vi "Main.vi"() -> ()   [LabVIEW 2018]
uses:
  C:/GIT/gaialabviewclient/Gaia_LabVIEW/Resources/JOT.GaiaClient.dll
  Gaia_LabVIEW/Resources/JOT.GaiaClient.dll
  Typedefs/States.ctl
  Typedefs/Element.ctl
  Typedefs/TestSequence.ctl
panel:
  out "EventLog":string="\r\n"
  out "ClientConnection":bool
  out "StateEnum":T1
  in  "baseUrl":string="http://172.23.225.64 "
  out "error out":errorcluster
  in  "Exit":bool
  in  "Tab Control":enum32{"TestSequense", "ManualControls"}(tab)
  in  "TestSeqMode":bool
  out "TestSequenceState":T2=enum."WaitDUT"
  in  "Recover":bool
  in  "Release":bool
  in  "Slide":bool
  in  "BatteryConnector":bool
  # "Stateful Applications"
  # "Triggers"
  # "More StateApp manual controls \ncan be added here"
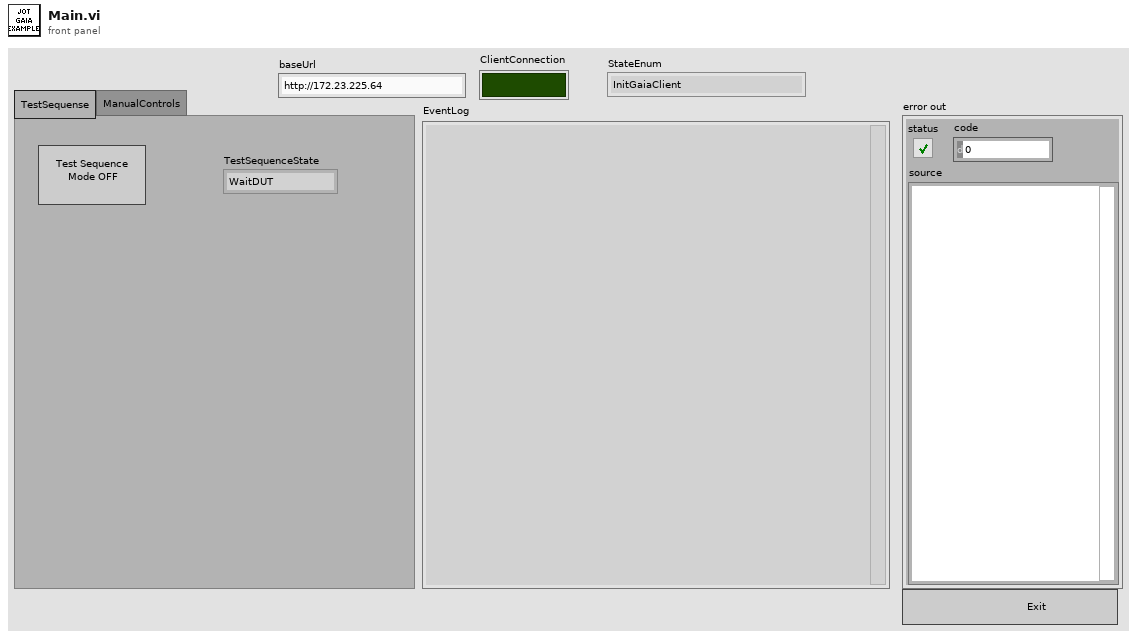
[diagram p1: front panel]
types:
  T1 = typedef "States.ctl" = enum16{"InitGaiaClient", "Idle", "AppsManualCtr", "StateTriggers", "TestSequence", "Exit"}
  T2 = typedef "TestSequence.ctl" = enum16{"SimulateDUTReplacement", "WaitDUT", "WaitReadyForTesting", "Test1", "ReleaseDUT"}
  T3 = typedef "Element.ctl" = cluster{"State":T1, "Application":string, "Action":string, "G code":string}
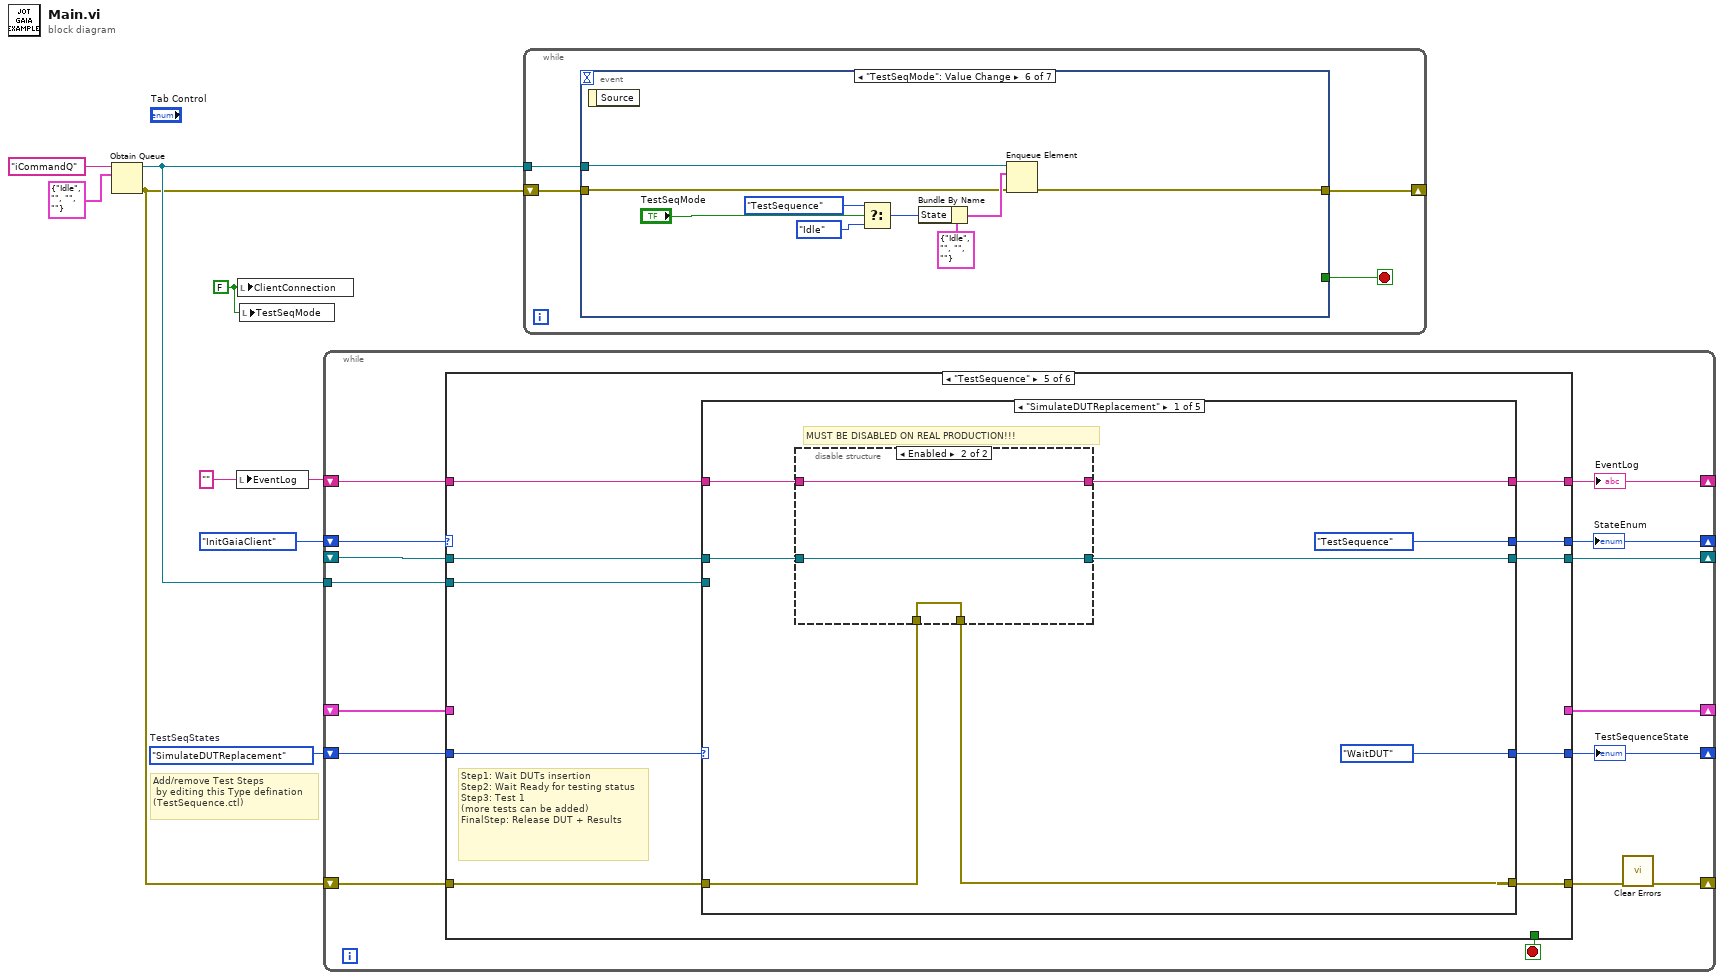
[diagram p0: block diagram]
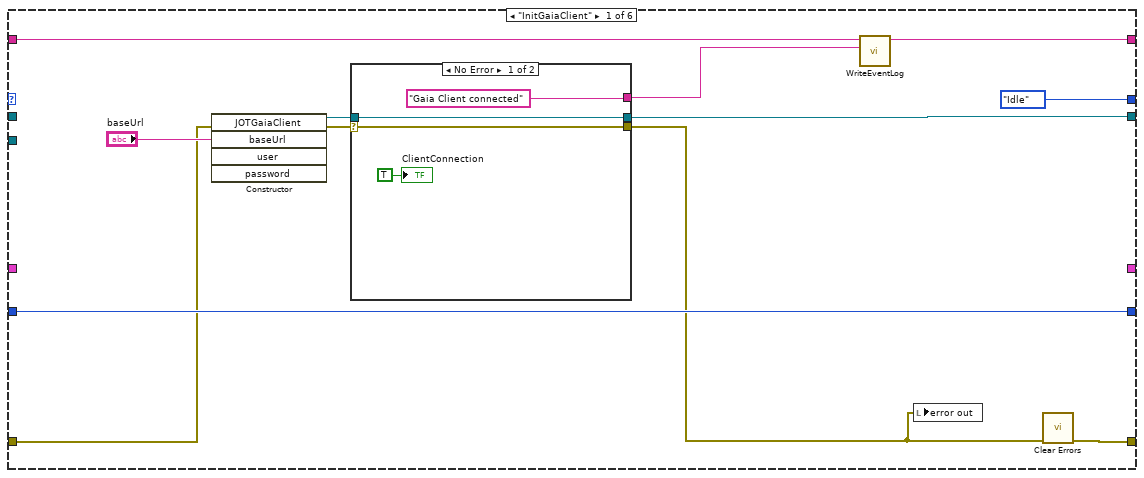
[diagram p2: hidden frame]
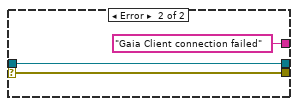
[diagram p3: hidden frame]
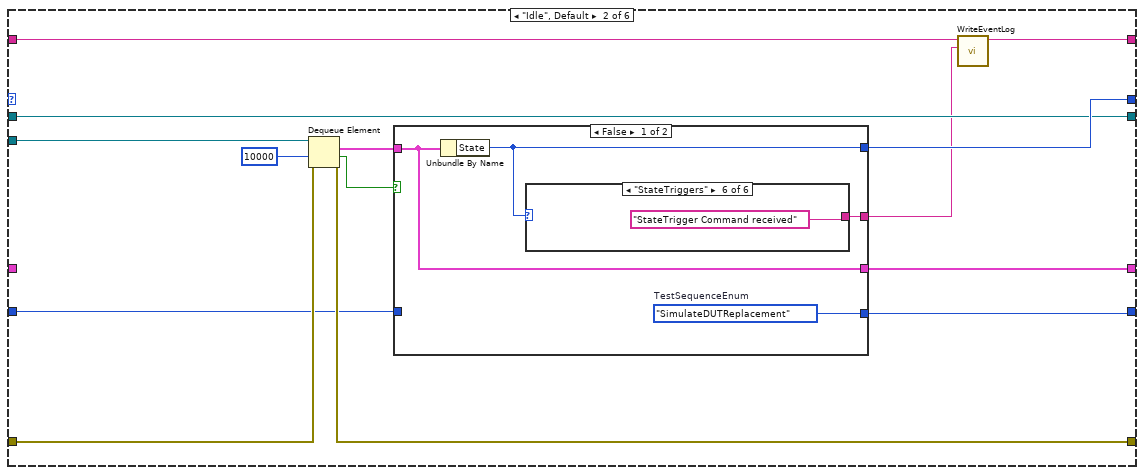
[diagram p4: hidden frame]
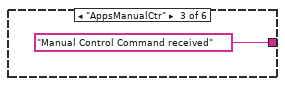
[diagram p7: hidden frame]
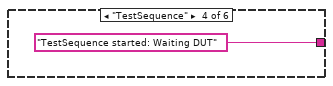
[diagram p8: hidden frame]
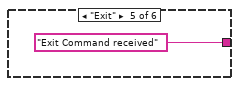
[diagram p9: hidden frame]
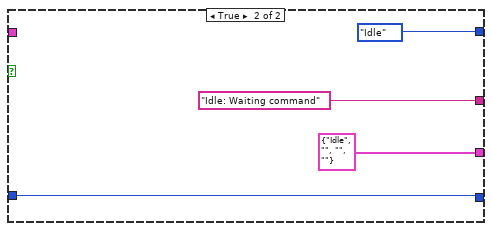
[diagram p10: hidden frame]
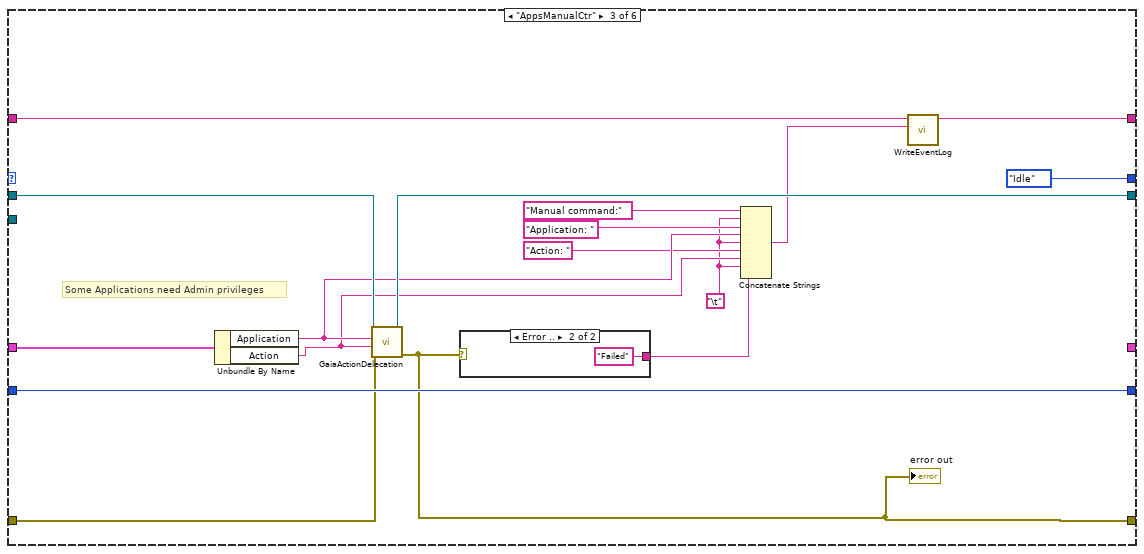
[diagram p11: hidden frame]
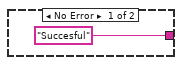
[diagram p12: hidden frame]
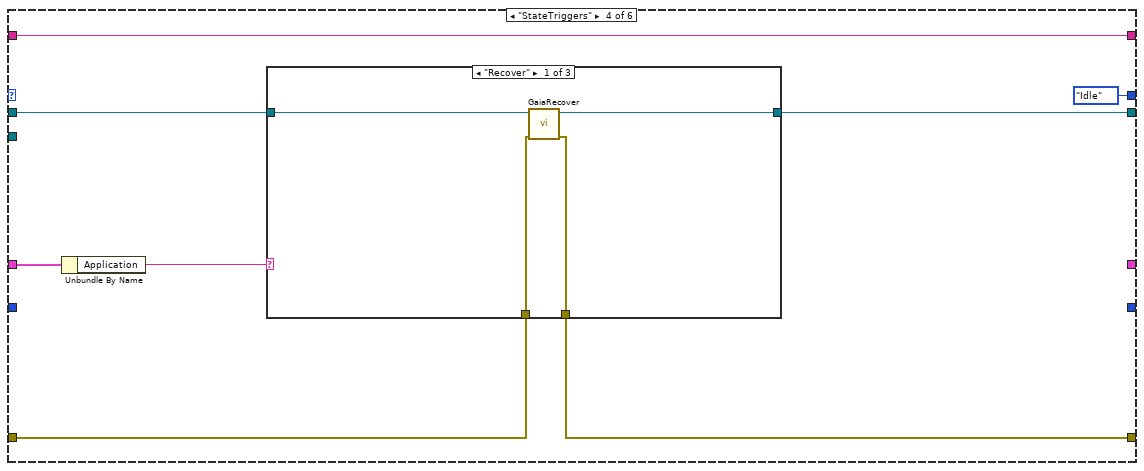
[diagram p13: hidden frame]
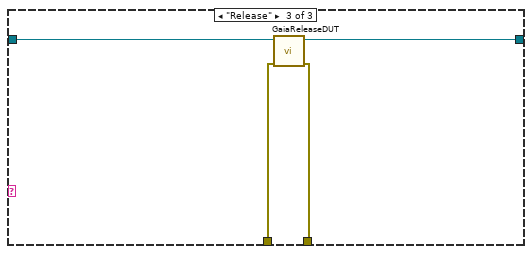
[diagram p15: hidden frame]
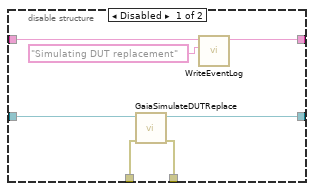
[diagram p16: hidden frame]
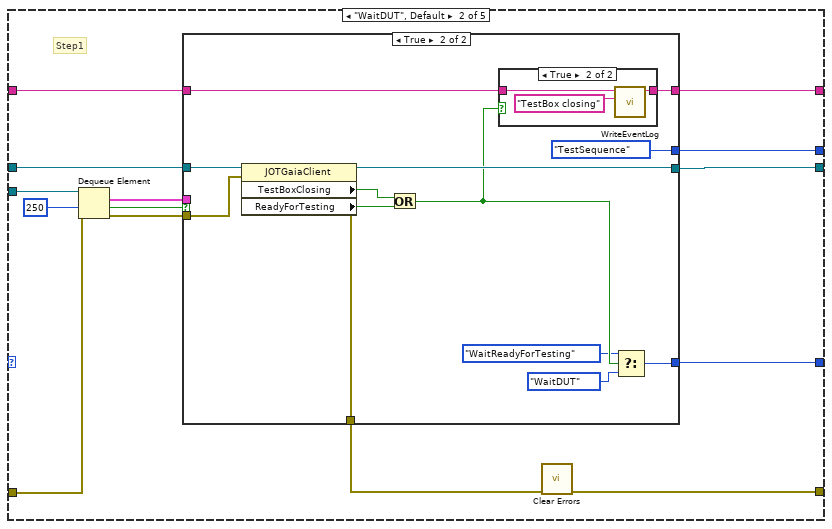
[diagram p17: hidden frame]
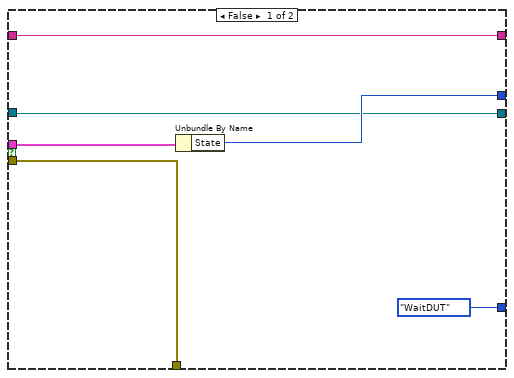
[diagram p18: hidden frame]
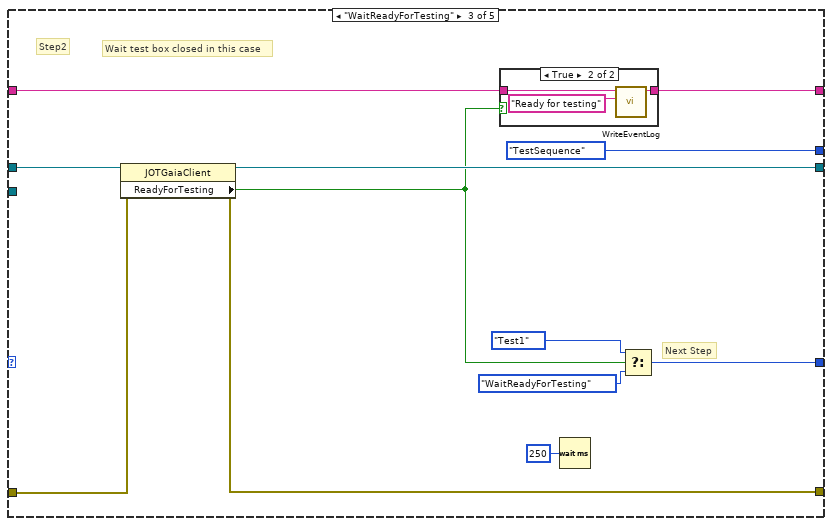
[diagram p20: hidden frame]
diagram:
  w1 = FALSE ("ClientConnection")
  w2 = ""
  w4 = TestSequence."SimulateDUTReplacement"  # TestSeqStates
  # "Add/remove Test Steps\n by editing this Type defination\n(TestSequence.ctl)"
  n1 = Obtain Queue(name (unnamed)="iCommandQ", element data type=T3 {"State"=enum."Idle", "Application"="", "Action"="", "G code"=""}) -> (queue out=w5:refnum<queue>, error out=w3:errorcluster)  [unwired: 3 in, 1 out]
  n2 = local write "EventLog"(w2) -> ()
  n3 = local write "ClientConnection"(w1) -> ()
  n4 = local write "TestSeqMode"(w1) -> ()
  n5 = while {
    shift-right: [w13] -> _
    shift-left: States."InitGaiaClient" -> [w23]
    shift-right: [w22] -> _
    shift-left: _ -> [w16]
    shift-right: [w10] -> _
    shift-left: w3 -> [w20]
    tunnel: w5 -> [w19]
    shift-right: [w18] -> _
    shift-left: _ -> [w17]
    shift-right: [w14] -> _
    shift-left: w4 -> [w15]
    shift-right: [w11] -> _
    shift-left: w2 -> [w12]
    stop <- w21 stop-if-true
    n6 = case shown="\"TestSequence\"" w23 {
      tunnel: [_ _ _ _ _ TRUE] -> w21
      tunnel: [w29 w49 w81 w89 w114 _] -> w22
      tunnel: w20 -> [w30 w54 w80 w93 w111 w224]
      tunnel: [w24 w55 w69 w91 w110 w218] -> w9
      tunnel: [States."Idle" w50 States."Idle" States."Idle" w108 States."Exit"] -> w13
      tunnel: w19 -> [_ w53 _ _ w109 w227]
      tunnel: [_ w48 _ _ _ _] -> w18
      tunnel: w17 -> [_ _ w84 w92 _ _]
      tunnel: w16 -> [_ w49 w82 w94 w115 w230]
      tunnel: w15 -> [w32 w46 w83 _ w113 w228]
      tunnel: [w32 w47 w83 _ w112 w228] -> w14
      tunnel: w12 -> [w28 w45 w79 w95 w107 w222]
      tunnel: [w27 w44 w78 w95 w106 w221] -> w11
      frame "InitGaiaClient" {
        n7 = constructor class="JOTGaiaClient"(error in=w30, "baseUrl"="baseUrl") -> (reference out=w34:refnum<k24>, error out=w31:errorcluster)  [unwired: 4 in, 4 out]
        n8 = case shown="No Error" w31 {
          selector: w31 -> [w37 w42]
          tunnel: w34 -> [w39 w41]
          tunnel: [w37 w42] -> w25
          tunnel: [w39 w41] -> w29
          tunnel: ["Gaia Client connected" ("LogText") "Gaia Client connection failed" ("LogText")] -> w26
          frame No Error {
            "ClientConnection" <- TRUE ("ClientConnection")
          }
          frame Error {
          }
        }
        n9 = call "WriteEventLog.vi"("LogText"=w26, "EventLog"=w28) -> ("EventLogOut"=w27:string)  [unwired: 9 in]
        n10 = local write "error out"(w25) -> ()
        n11 = call <vilib>:"Clear Errors.vi"("error in (no error)"=w25) -> ("error out"=w24:errorcluster)  [unwired: 5 in, 1 out]
      }
      frame "Idle", Default {
        n12 = Dequeue Element(queue=w53, timeout in ms (-1)=10000, error in (no error)=w54) -> (element=w56:T3, timed out?=w51:bool, error out=w55:errorcluster)  [unwired: 1 out]
        n13 = case shown="False" w51 {
          tunnel: w56 -> [w60 _]
          tunnel: [w58 States."Idle"] -> w50
          tunnel: [w60 T3 {"State"=enum."Idle", "Application"="", "Action"="", "G code"=""}] -> w48
          tunnel: [w59 w66] -> w47
          tunnel: w46 -> [_ w66]
          tunnel: [w57 "Idle: Waiting command" ("LogText")] -> w43
          frame False {
            w59 = TestSequence."SimulateDUTReplacement"  # TestSequenceEnum
            n14 = Unbundle By Name(w60) -> ("State"=w58:T1)
            n15 = case shown="\"StateTriggers\"" w58 {
              tunnel: [_ _ "Manual Control Command received" "TestSequence started: Waiting DUT" "Exit Command received" "StateTrigger Command received"] -> w57
              frame "InitGaiaClient", Default {
              }
              frame "Idle" {
              }
              frame "AppsManualCtr" {
              }
              frame "TestSequence" {
              }
              frame "Exit" {
              }
              frame "StateTriggers" {
              }
            }
          }
          frame True {
          }
        }
        n16 = call "WriteEventLog.vi"("LogText"=w43, "EventLog"=w45) -> ("EventLogOut"=w44:string)  [unwired: 9 in]
      }
      frame "AppsManualCtr" {
        w70 = "\t"
        # "Some Applications need Admin privileges"
        n17 = Unbundle By Name(w84) -> ("Application"=w77:string, "Action"=w76:string)
        n18 = call "GaiaActionDelecation.vi"("Error in"=w80, "Action"=w76, "Application"=w77, "ClientRef"=w82) -> ("error out"=w69:errorcluster, "ClientRef out"=w81:refnum<k24>)  [unwired: 6 in]
        "error out" <- w69
        n19 = case shown="Error .." w69 {
          tunnel: ["Succesful" ("string") "Failed" ("string")] -> w71
          frame No Error {
          }
          frame Error {
          }
        }
        n20 = Concatenate Strings("Manual command:" ("string"), w70, "Application: " ("string"), w77, w70, "Action: " ("string"), w76, w70, w71) -> (w72:string)
        n21 = call "WriteEventLog.vi"("LogText"=w72, "EventLog"=w79) -> ("EventLogOut"=w78:string)  [unwired: 9 in]
      }
      frame "StateTriggers" {
        n22 = Unbundle By Name(w92) -> ("Application"=w90:string)
        n23 = case shown="\"Recover\"" w90 {
          tunnel: w94 -> [w97 w101 w105]
          tunnel: w93 -> [w99 w100 w104]
          tunnel: [w98 w100 w103] -> w91
          tunnel: [w96 w101 w102] -> w89
          frame "Recover" {
            n24 = call "GaiaRecover.vi"("error in (no error)"=w99, ".NET Refnum in"=w97) -> ("error out"=w98:errorcluster, ".NET Refnum out"=w96:refnum<k24>)  [unwired: 8 in]
          }
          frame "None", Default {
          }
          frame "Release" {
            n25 = call "GaiaReleaseDUT.vi"("error in (no error)"=w104, ".NET Refnum in"=w105) -> ("error out"=w103:errorcluster, ".NET Refnum out"=w102:refnum<k24>)  [unwired: 8 in]
          }
        }
      }
      frame "TestSequence" {
        # "Step1: Wait DUTs insertion \nStep2: Wait Ready for testing status\nStep3: Test 1\n(more tests can be added)\nFinalStep: Release DUT + Results"
        n26 = case shown="\"SimulateDUTReplacement\"" w113 {
          tunnel: w115 -> [w121 w137 w182 w198 w215]
          tunnel: [w120 w147 w175 w188 w211] -> w114
          tunnel: [TestSequence."WaitDUT" w146 w179 TestSequence."ReleaseDUT" TestSequence."SimulateDUTReplacement"] -> w112
          tunnel: w111 -> [w119 w142 w177 w196 w210]
          tunnel: [w118 w138 w176 w190 w209] -> w110
          tunnel: w109 -> [_ w143 _ _ _]
          tunnel: [States."TestSequence" w141 States."TestSequence" States."TestSequence" States."TestSequence"] -> w108
          tunnel: w107 -> [w123 w135 w173 w194 w213]
          tunnel: [w122 w134 w172 w192 w212] -> w106
          frame "SimulateDUTReplacement" {
            # "MUST BE DISABLED ON REAL PRODUCTION!!!"
            n27 = disable-structure shown="Enabled" {
              disable-tunnel: w123 -> [w130 w133]
              disable-tunnel: [w129 w133] -> w122
              disable-tunnel: w121 -> [w127 w132]
              disable-tunnel: [w126 w132] -> w120
              disable-tunnel: w119 -> [w125 w131]
              disable-tunnel: [w124 w131] -> w118
              frame Disabled {
                n28 = call "GaiaSimulateDUTReplace.vi"("error in"=w125, "GaiaClientRef in"=w127) -> ("error out"=w124:errorcluster, "GaiaClientRef out"=w126:refnum<k24>)  [unwired: 8 in]
                n29 = call "WriteEventLog.vi"("LogText"="Simulating DUT replacement", "EventLog"=w130) -> ("EventLogOut"=w129:string)  [unwired: 9 in]
              }
              frame Enabled {
              }
            }
          }
          frame "WaitDUT", Default {
            # "Step1"
            n30 = Dequeue Element(queue=w143, timeout in ms (-1)=250, error in (no error)=w142) -> (element=w139:T3, timed out?=w140:bool, error out=w136:errorcluster)  [unwired: 1 out]
            n31 = case shown="True" w140 {
              tunnel: [w150 w166] -> w147
              tunnel: [TestSequence."WaitDUT" w163] -> w146
              tunnel: [w149 w162] -> w145
              tunnel: [w151 States."TestSequence"] -> w141
              tunnel: w139 -> [w152 _]
              tunnel: w137 -> [w150 w159]
              tunnel: w136 -> [w149 w160]
              tunnel: w135 -> [w148 w158]
              tunnel: [w148 w157] -> w134
              frame False {
                n32 = Unbundle By Name(w152) -> ("State"=w151:T1)
              }
              frame True {
                n33 = property class="JOTGaiaClient"(reference=w159, error in=w160) -> (reference out=w166:refnum<k24>, error out=w162:errorcluster, "TestBoxClosing"=w165:bool, "ReadyForTesting"=w164:bool)
                n34 = Or(x=w165, y=w164) -> (x .or. y?=w156:bool)
                n35 = case shown="True" w156 {
                  tunnel: w158 -> [w167 w170]
                  tunnel: [w167 w168] -> w157
                  frame False {
                  }
                  frame True {
                    n36 = call "WriteEventLog.vi"("LogText"="TestBox closing", "EventLog"=w170) -> ("EventLogOut"=w168:string)  [unwired: 9 in]
                  }
                }
                n37 = Select(t=TestSequence."WaitReadyForTesting", s=w156, f=TestSequence."WaitDUT") -> (s? t:f=w163:T2)
              }
            }
            n38 = call <vilib>:"Clear Errors.vi"("error in (no error)"=w145) -> ("error out"=w138:errorcluster)  [unwired: 5 in, 1 out]
          }
          frame "WaitReadyForTesting" {
            # "Next Step"
            # "Step2"
            # "Wait test box closed in this case"
            n39 = property class="JOTGaiaClient"(reference=w182, error in=w177) -> (reference out=w175:refnum<k24>, error out=w176:errorcluster, "ReadyForTesting"=w171:bool)
            n40 = case shown="True" w171 {
              tunnel: w173 -> [w183 w186]
              tunnel: [w183 w184] -> w172
              frame False {
              }
              frame True {
                n41 = call "WriteEventLog.vi"("LogText"="Ready for testing", "EventLog"=w186) -> ("EventLogOut"=w184:string)  [unwired: 9 in]
              }
            }
            n42 = Wait (ms)(milliseconds to wait=u32 250) -> ()  [unwired: 1 out]
            n43 = Select(t=TestSequence."Test1", s=w171, f=TestSequence."WaitReadyForTesting") -> (s? t:f=w179:T2)
          }
          frame "Test1" {
            w191 = "MainRobot" ("Application")
            # "Options for G-code reading:\nConstant, Variable, file"
            # "Step3"
            # "Nest Step"
            # "Run G-code example"
            n44 = call "WriteEventLog.vi"("LogText"="G-Code test started", "EventLog"=w194) -> ("EventLogOut"=w192:string)  [unwired: 9 in]
            n45 = call "GaiaActionDelecation.vi"("plainText"="N000 F50 E500 E-500\nN001 G17\n\nN005 G01 X72.976 Y55.977 Z-0.128\nN010 G01 X198.252 Y56.442 Z-0.128\nN015 G01 X198.234 Y162.025 Z-0.128\nN020 G01 X85.468 Y162.026 Z-0.128\nN025 G01 X85.411 Y94.005 Z-0.128\nN030 G01 X85.411 Y94.005 Z7.940\nN035 G01 X85.411 Y94.005 Z-0.124", "Error in"=w196, "Action"="cnc_run", "Application"=w191, "ClientRef"=w198) -> ("error out"=w187:errorcluster, "ClientRef out"=w189:refnum<k24>)  [unwired: 5 in]
            n46 = local write "EventLog"(w192) -> ()
            n47 = case shown="No Error" w187 {
              selector: w187 -> [w201 w207]
              tunnel: w191 -> [w206 _]
              tunnel: [w205 w207] -> w190
              tunnel: w189 -> [w204 w208]
              tunnel: [w203 w208] -> w188
              frame No Error {
                n48 = call "GaiaActionWaitStateReady.vi"("Error in"=w201, "Timeout"=20000, "Application"=w206, "ClientRef"=w204) -> ("error out"=w205:errorcluster, "ClientRef out"=w203:refnum<k24>)  [unwired: 6 in]
              }
              frame Error {
                n49 = local write "error out"(w207) -> ()
              }
            }
          }
          frame "ReleaseDUT" {
            # "Stay in Test sequence mode"
            # "Back to first Step"
            # "Final Step\nRelease DUT"
            n50 = call "GaiaReleaseDUT.vi"("error in (no error)"=w210, ".NET Refnum in"=w215) -> ("error out"=w209:errorcluster, ".NET Refnum out"=w211:refnum<k24>)  [unwired: 8 in]
            n51 = call "WriteEventLog.vi"("LogText"="DUT released", "EventLog"=w213) -> ("EventLogOut"=w212:string)  [unwired: 9 in]
          }
        }
      }
      frame "Exit" {
        w219 = FALSE ("ClientConnection")
        n52 = Flush Queue(queue=w227, error in (no error)=w224) -> (queue out=w226:refnum<queue>, error out=w225:errorcluster)  [unwired: 1 out]
        n53 = Release Queue(queue=w226, error in (no error)=w225) -> (error out=w223:errorcluster)  [unwired: 1 in, 2 out]
        n54 = Close Reference(reference=w230, error in (no error)=w223) -> (error out=w218:errorcluster)
        n55 = local write "ClientConnection"(w219) -> ()
        n56 = local write "TestSeqMode"(w219) -> ()
        n57 = call "WriteEventLog.vi"("LogText"="SW exit", "EventLog"=w222) -> ("EventLogOut"=w221:string)  [unwired: 9 in]
      }
    }
    "TestSequenceState" <- w14
    "StateEnum" <- w13
    "EventLog" <- w11
    n58 = call <vilib>:"Clear Errors.vi"("error in (no error)"=w9) -> ("error out"=w10:errorcluster)  [unwired: 5 in, 1 out]
  }
  n59 = while {
    tunnel: w5 -> [w235]
    shift-right: [w234] -> _
    shift-left: w3 -> [w233]
    stop <- w232 stop-if-true
    n60 = event shown="[5] \"TestSeqMode\": Value Change" {
      selector: _ -> [_ _ _ _ _ _ _]
      dyn-events: _ -> [_ _ _ _ _ _ _]
      timeout: _ -> [_ _ _ _ _ _ _]
      tunnel: w235 -> [_ w240 w258 w265 w272 w278 w284]
      tunnel: [w236 w237 w249 w260 w268 w279 w282] -> w234
      tunnel: w233 -> [w236 w239 w248 w259 w267 w277 w283]
      tunnel: [_ _ _ _ _ _ TRUE] -> w232
      event Timeout {
        n61 = event-data() -> ()  [unwired: 1 in, 3 out]
      }
      event "BatteryConnector": Value Change {
        n62 = event-data() -> ()  [unwired: 1 in, 1 out]
        n63 = Select(t="set-Home" ("key"), s="BatteryConnector", f="set-Work" ("key")) -> (s? t:f=w243:string)
        n64 = Bundle By Name(cluster=T3 {"State"=enum."Idle", "Application"="", "Action"="", "G code"=""}, "State"=States."AppsManualCtr", "Application"="BatteryConnector", "Action"=w243) -> (w246:T3)
        n65 = Enqueue Element(queue=w240, element=w246, error in (no error)=w239) -> (error out=w237:errorcluster)  [unwired: 1 in, 2 out]
      }
      event "Slide": Value Change {
        # "Slide need Admin privileges"
        n66 = event-data() -> ()  [unwired: 1 in, 1 out]
        n67 = Select(t="set-Open" ("key"), s="Slide", f="set-Close" ("key")) -> (s? t:f=w252:string)
        n68 = Bundle By Name(cluster=T3 {"State"=enum."Idle", "Application"="", "Action"="", "G code"=""}, "State"=States."AppsManualCtr", "Application"="Slide", "Action"=w252) -> (w256:T3)
        n69 = Enqueue Element(queue=w258, element=w256, error in (no error)=w248) -> (error out=w249:errorcluster)  [unwired: 1 in, 2 out]
      }
      event "Release": Mouse Down {
        n70 = event-data() -> ()  [unwired: 1 in, 8 out]
        n71 = Bundle By Name(cluster=T3 {"State"=enum."Idle", "Application"="", "Action"="", "G code"=""}, "State"=States."StateTriggers", "Application"="Release") -> (w263:T3)
        n72 = Enqueue Element(queue=w265, element=w263, error in (no error)=w259) -> (error out=w260:errorcluster)  [unwired: 1 in, 2 out]
      }
      event "Recover": Mouse Down {
        n73 = event-data() -> ()  [unwired: 1 in, 8 out]
        n74 = Bundle By Name(cluster=T3 {"State"=enum."Idle", "Application"="", "Action"="", "G code"=""}, "State"=States."StateTriggers", "Application"="Recover") -> (w270:T3)
        n75 = Enqueue Element(queue=w272, element=w270, error in (no error)=w267) -> (error out=w268:errorcluster)  [unwired: 1 in, 2 out]
      }
      event "TestSeqMode": Value Change {
        n76 = event-data() -> ()  [unwired: 1 in, 1 out]
        n77 = Select(t=States."TestSequence" ("State"), s="TestSeqMode", f=States."Idle" ("State")) -> (s? t:f=w273:T1)
        n78 = Bundle By Name(cluster=T3 {"State"=enum."Idle", "Application"="", "Action"="", "G code"=""}, "State"=w273) -> (w280:T3)
        n79 = Enqueue Element(queue=w278, element=w280, error in (no error)=w277) -> (error out=w279:errorcluster)  [unwired: 1 in, 2 out]
      }
      event "Exit": Mouse Down {
        n80 = event-data() -> ()  [unwired: 1 in, 1 out]
        n81 = Bundle By Name(cluster=T3 {"State"=enum."Idle", "Application"="", "Action"="", "G code"=""}, "State"=States."Exit") -> (w286:T3)
        n82 = Enqueue Element(queue=w284, element=w286, error in (no error)=w283) -> (error out=w282:errorcluster)  [unwired: 1 in, 2 out]
      }
    }
  }
